vi "SwerveKinematics.vi"(8 "Rotation Center Choice":T1(ring), 9 "Joystick Rotation":dbl(slide) scale=1.0..-1.0, 10 "Joystick Y":dbl(slide) scale=1.0..-1.0, 11 "Joystick X":dbl(slide) scale=-1.0..1.0) -> (0 "Module 3 Velocity Command (ul)":dbl(slide) scale=0.0..1.0 scale format="%.2f", 1 "Module 2 Velocity Command (ul)":dbl(slide) scale=0.0..1.0 scale format="%.2f", 2 "Module 1 Velocity Command (ul)":dbl(slide) scale=0.0..1.0 scale format="%.2f", 3 "Module 0 Velocity Command (ul)":dbl(slide) scale=0.0..1.0 scale format="%.2f", 4 "Module 2 Angle (deg)":dbl(knob) scale=180.0..-180.0 scale format="%#_6f", 5 "Module 1 Angle (deg)":dbl(knob) scale=180.0..-180.0 scale format="%#_6f", 6 "Module 3 Angle (deg)":dbl(knob) scale=180.0..-180.0 scale format="%#_6f", 7 "Module 0 Angle (deg)":dbl(knob) scale=180.0..-180.0 scale format="%#_6f")   [LabVIEW 2019]
doc: "Performs the kinematics for a rectangular four wheel swerve robot with a selectable center of rotation. Swerve module #0 is located in the front right corner and the modules increment in the counter-clockwise direction."
panel:
  in  "Robot Width (in)":dbl=25.0
  in  "Robot Length (in)":dbl=25.0
  # "\"Front\" of Robot"
  # "M1"
  # "M0"
  # "Left Thumbstick"
  # "Right Thumbstick"
  # "X"
  # "Y"
  # "(0,0)"
  # "+CCW"
  # "M2"
  # "M3"
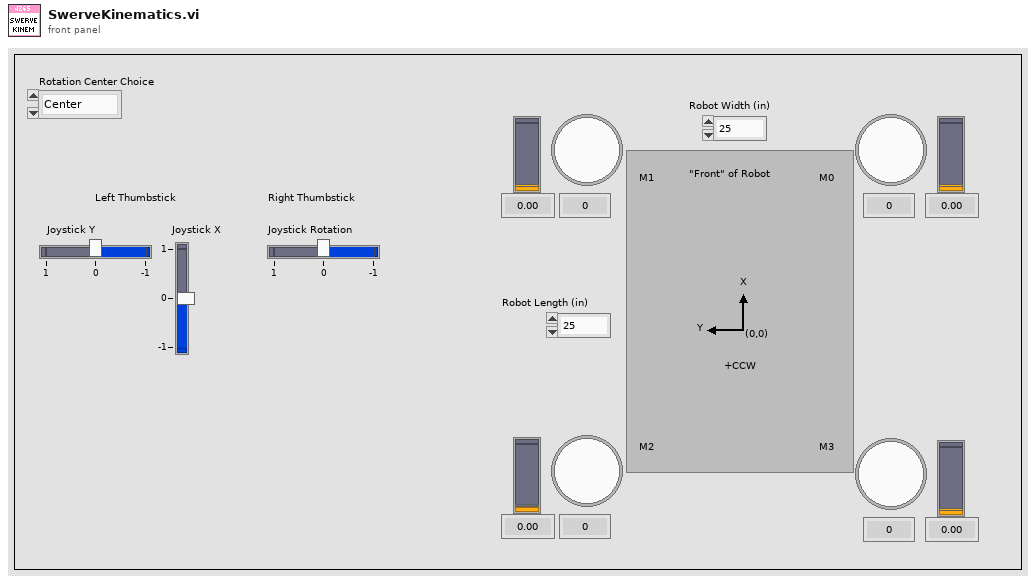
[diagram p1: front panel]
types:
  T1 = enum16{"Center", "Module 0", "Module 1", "Module 2", "Module 3"}
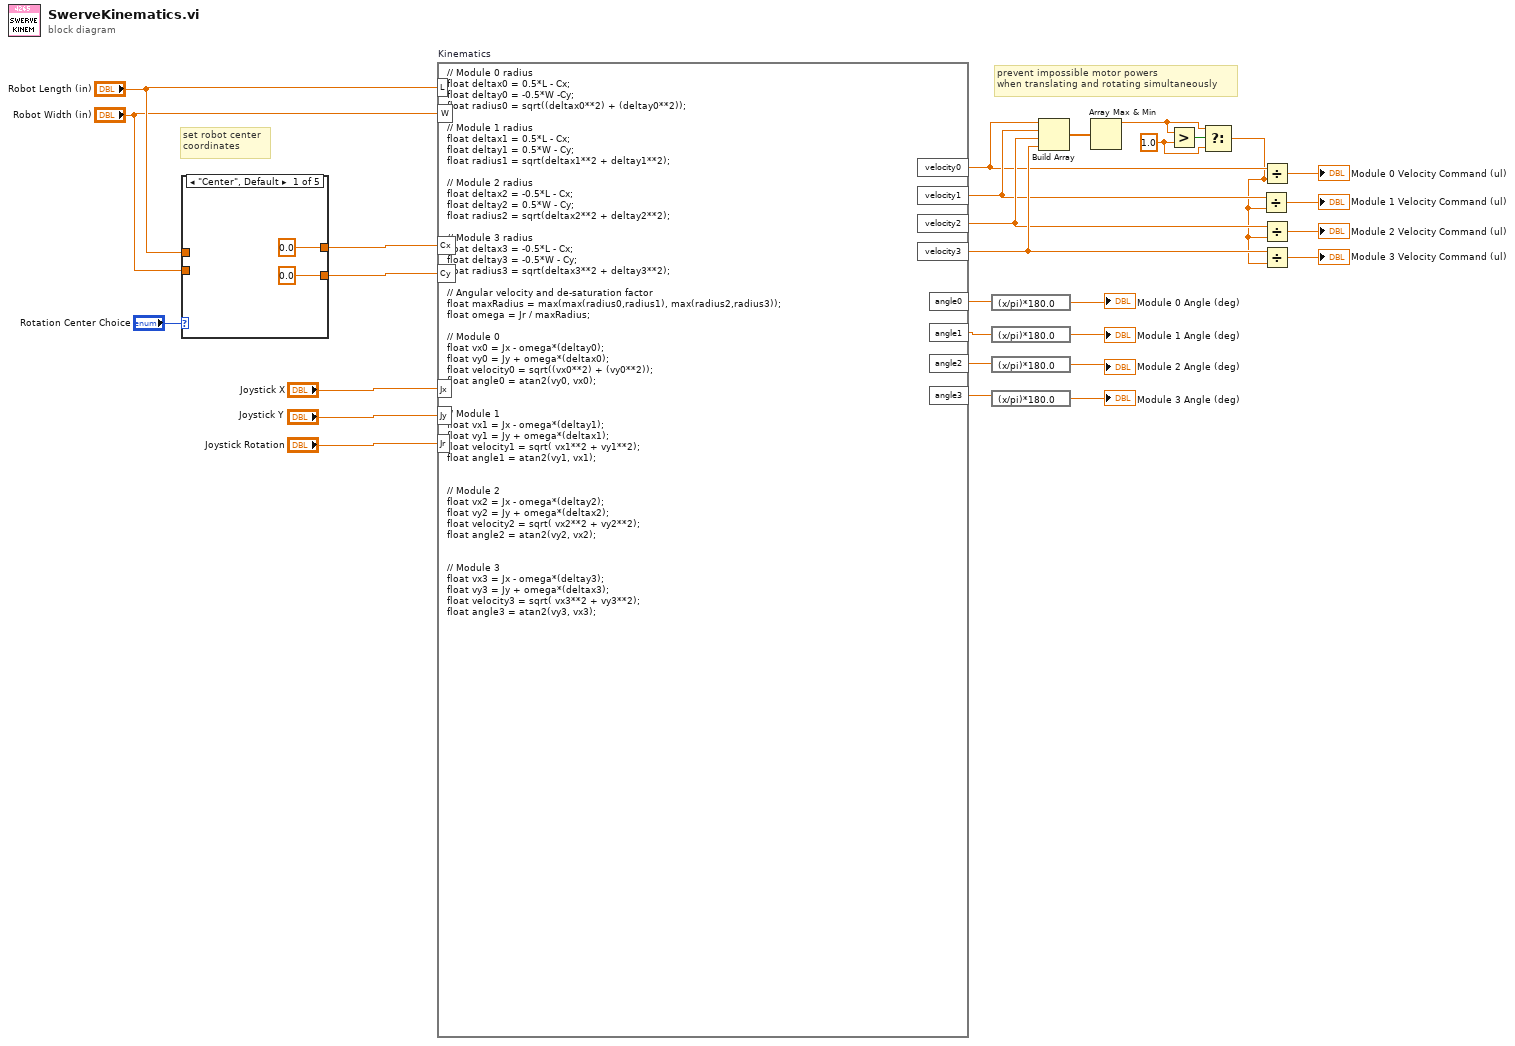
[diagram p0: block diagram]
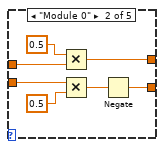
[diagram p2: hidden frame]
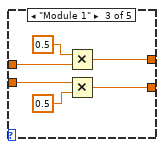
[diagram p3: hidden frame]
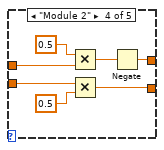
[diagram p4: hidden frame]
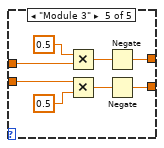
[diagram p5: hidden frame]
diagram:
  w16 = 1.0 ("y")
  # "prevent impossible motor powers\nwhen translating and rotating simultaneously"
  # "set robot center \ncoordinates"
  n1 = case shown="\"Center\", Default" "Rotation Center Choice" {
    tunnel: [0.0 w37 w40 w46 w53] -> w25
    tunnel: [0.0 w32 w39 w45 w52] -> w24
    tunnel: "Robot Length (in)" -> [_ w38 w42 w49 w57]
    tunnel: "Robot Width (in)" -> [_ w35 w41 w48 w56]
    frame "Center", Default {
    }
    frame "Module 0" {
      n2 = Multiply(x=0.5, y=w38) -> (x*y=w37:dbl)
      n3 = Multiply(x=w35, y=0.5) -> (x*y=w34:dbl)
      n4 = Negate(x=w34) -> (-x=w32:dbl)
    }
    frame "Module 1" {
      n5 = Multiply(x=0.5, y=w42) -> (x*y=w40:dbl)
      n6 = Multiply(x=w41, y=0.5) -> (x*y=w39:dbl)
    }
    frame "Module 2" {
      n7 = Multiply(x=0.5, y=w49) -> (x*y=w47:dbl)
      n8 = Multiply(x=w48, y=0.5) -> (x*y=w45:dbl)
      n9 = Negate(x=w47) -> (-x=w46:dbl)
    }
    frame "Module 3" {
      n10 = Multiply(x=0.5, y=w57) -> (x*y=w55:dbl)
      n11 = Multiply(x=w56, y=0.5) -> (x*y=w54:dbl)
      n12 = Negate(x=w55) -> (-x=w53:dbl)
      n13 = Negate(x=w54) -> (-x=w52:dbl)
    }
  }
  n14 = formula code="// Module 0 radius\nfloat deltax0 = 0.5*L - Cx;\nfloat deltay0 = -0.5*W -Cy; \nfloat radius0 = sqrt((deltax0**2) + (deltay0**2));\n\n// Module 1 radius\nfloat deltax1 = 0.5*L - Cx;\nfloat deltay1 = 0.5*W - Cy;\nfloat radius1 = sqrt(deltax1**2 + deltay1**2);\n\n// Module 2 radius\nfloat deltax2 = -0.5*L - Cx;\nfloat deltay2 = 0.5*W - Cy;\nfloat radius2 = sqrt(deltax2**2 + deltay2**2);\n\n// Module 3 radius\nfloat deltax3 = -0.5*L - Cx;\nfloat deltay3 = -0.5*W - Cy;\nfloat radius3 = sqrt(deltax3**2 + deltay3**2);\n\n// Angular velocity and de-saturation factor\nfloat maxRadius = max(max(radius0,radius1), max(radius2,radius3));\nfloat omega = Jr / maxRadius;\n\n// Module 0\nfloat vx0 = Jx - omega*(deltay0);\nfloat vy0 = Jy + omega*(deltax0);\nfloat velocity0 = sqrt((vx0**2) + (vy0**2));\nfloat angle0 = atan2(vy0, vx0);\n\n\n// Module 1\nfloat vx1 = Jx - omega*(deltay1);\nfloat vy1 = Jy + omega*(deltax1);\nfloat velocity1 = sqrt( vx1**2 + vy1**2);\nfloat angle1 = atan2(vy1, vx1);\n\n\n// Module 2\nfloat vx2 = Jx - omega*(deltay2);\nfloat vy2 = Jy + omega*(deltax2);\nfloat velocity2 = sqrt( vx2**2 + vy2**2);\nfloat angle2 = atan2(vy2, vx2);\n\n\n// Module 3\nfloat vx3 = Jx - omega*(deltay3);\nfloat vy3 = Jy + omega*(deltax3);\nfloat velocity3 = sqrt( vx3**2 + vy3**2);\nfloat angle3 = atan2(vy3, vx3);" "Kinematics"("L"="Robot Length (in)", "W"="Robot Width (in)", "Cx"=w25, "Cy"=w24, "Jr"="Joystick Rotation", "Jx"="Joystick X", "Jy"="Joystick Y") -> ("velocity0"=w10:dbl, "angle0"=w27:dbl, "angle1"=w20:dbl, "angle2"=w19:dbl, "angle3"=w18:dbl, "velocity1"=w11:dbl, "velocity2"=w12:dbl, "velocity3"=w13:dbl)
  n15 = expression code="(x/pi)*180.0" ("radians to degrees")(w27) -> (→"Module 0 Angle (deg)":dbl)
  n16 = expression code="(x/pi)*180.0" ("radians to degrees")(w20) -> (→"Module 1 Angle (deg)":dbl)
  n17 = expression code="(x/pi)*180.0" ("radians to degrees")(w19) -> (→"Module 2 Angle (deg)":dbl)
  n18 = expression code="(x/pi)*180.0" ("radians to degrees")(w18) -> (→"Module 3 Angle (deg)":dbl)
  n19 = Build Array(w10, w11, w12, w13) -> (w14:dbl[])
  n20 = Array Max & Min(array=w14) -> (max value=w15:dbl)  [unwired: 3 out]
  n21 = Greater?(x=w15, y=w16) -> (0:w17:bool)
  n22 = Select(t=w15, s=w17, f=w16) -> (s? t:f=w1:dbl)
  n23 = Divide(x=w11, y=w1) -> (x/y=→"Module 1 Velocity Command (ul)":dbl)
  n24 = Divide(x=w10, y=w1) -> (x/y=→"Module 0 Velocity Command (ul)":dbl)
  n25 = Divide(x=w12, y=w1) -> (x/y=→"Module 2 Velocity Command (ul)":dbl)
  n26 = Divide(x=w13, y=w1) -> (x/y=→"Module 3 Velocity Command (ul)":dbl)
